vi "Get Robot Response.vi"(8 "error in (no error)":errorcluster, 11 "UR5 Robot in":refnum<class "UR5 Robot.lvclass">) -> (0 "error out":errorcluster, 2 "Status":string, 3 "UR5 Robot out":refnum<class "UR5 Robot.lvclass">)   [LabVIEW 2018, in "UR5 Robot.lvlib" / "UR5 Robot.lvclass"]
uses:
  UR5 Robot.lvclass
  UR5 Robot.lvclass/UR5 Robot.ctl
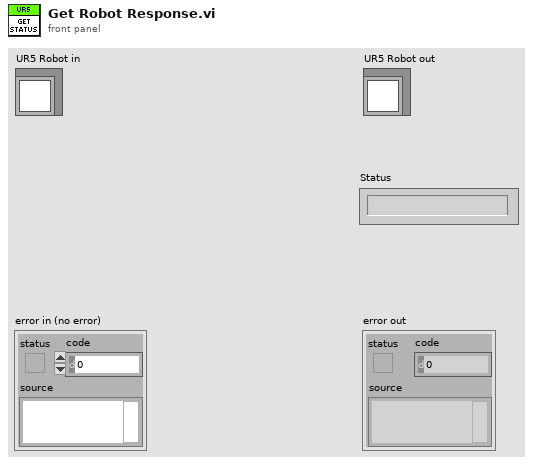
[diagram p1: front panel]
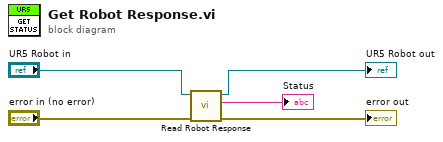
[diagram p0: block diagram]
diagram:
  n1 = call "Read Robot Response.vi"("error in (no error)"="error in (no error)", "UR5 Robot in"="UR5 Robot in") -> ("error out"=→"error out":errorcluster, "Robot Response"=→"Status":string, "UR5 Robot out"=→"UR5 Robot out":refnum<class "UR5 Robot.lvclass">)  [unwired: 7 in]
